vi "Set value by string.vi"(8 "error in (no error)":errorcluster, 10 "Value":string, 11 "Column in":refnum<class "Text Field.lvclass">) -> (0 "error out":errorcluster, 3 "Column out":refnum<class "Text Field.lvclass">)   [LabVIEW 2020]
uses:
  Text Field.lvclass
  Basic Fields/Basic Field Class/Ctrl Refnum Column.lvclass
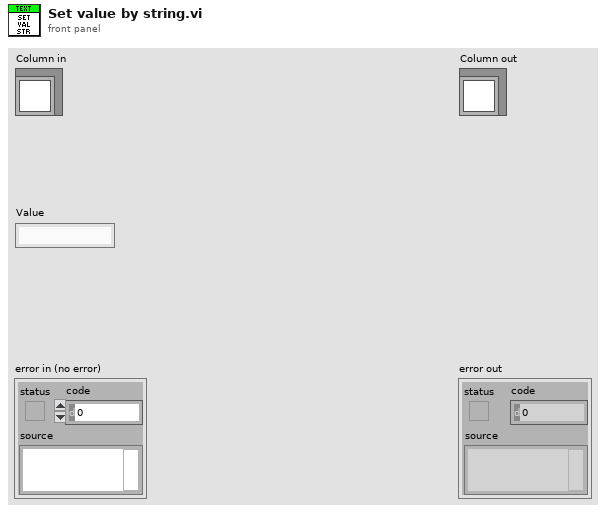
[diagram p1: front panel]
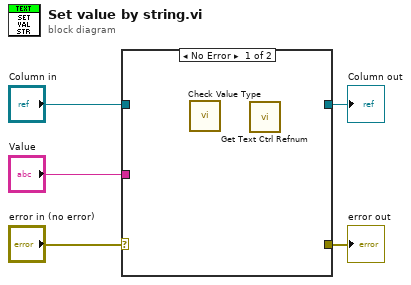
[diagram p0: block diagram]
diagram:
  n1 = case shown="No Error" "error in (no error)" {
    selector: "error in (no error)" -> [_ w7]
    tunnel: [_ w7] -> w4
    tunnel: "Column in" -> [_ w6]
    tunnel: [_ w6] -> w2
    tunnel: "Value" -> [_ _]
    frame No Error {
      n2 = call-dynamic "Check Value Type.vi"() -> ()  [unwired: 10 in, 2 out]
      n3 = call "Get Text Ctrl Refnum.vi"() -> ()  [unwired: 9 in, 3 out]
    }
    frame Error {
    }
  }
  "error out" <- w4
  "Column out" <- w2
